vi "AIT 1553 Main Page.vi"(8 "error in (no error)":errorcluster, 11 "Node Ptr":T1 format="%.0x") -> (0 "error out":errorcluster)   [LabVIEW 2015, in "AIT 1553 Custom Device.lvlib"]
uses:
  AIT 1553 Custom Device.lvlib
  <vilib>/NI Veristand/Custom Device API/Custom Device Item Ref.ctl
  Controls and Global/Global.vi
  <vilib>/NI Veristand/Custom Device API/Set Item Property (Boolean).vi
  <vilib>/NI Veristand/Custom Device API/Get Item Property (U16).vi
  <vilib>/NI Veristand/Custom Device API/Get Item Property (Variant).vi
  <vilib>/NI Veristand/Custom Device API/Set Item Property (Variant).vi
  <vilib>/NI Veristand/Custom Device API/Set Item Property (U16).vi
  <vilib>/NI Veristand/Custom Device API/Custom Device API.lvlib
panel:
  in  "Board Index (0 Based)":u16
  in  "Bus 4":bool
  in  "Bus 3":bool
  in  "Bus 2":bool
  in  "Bus 1":bool
  out "Version":string
  in  "Board Serial #":u64
  in  "Header":cluster{"Section Name":string}={"Section Name"="AIT 1553 Device"}
  in  "Description":string
  in  "Name":string
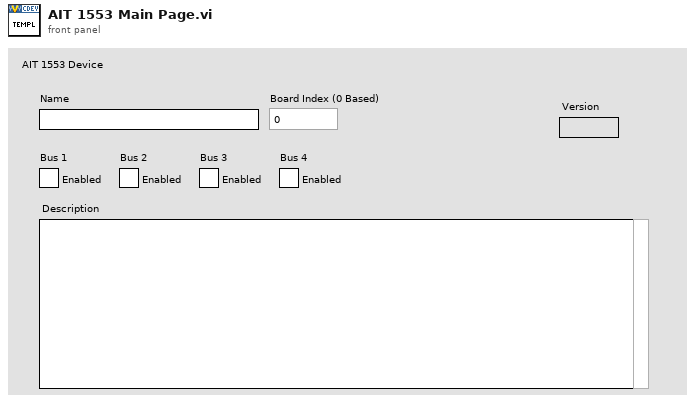
[diagram p1: front panel]
types:
  T1 = typedef "Custom Device API.lvlib/Custom Device Item Ref.ctl" = u64
  T2 = typedef "AIT 1553 Custom Device.lvlib/1553 Bus Enabled.ctl" = cluster{"Bus1Enabled":bool, "Bus2Enabled":bool, "Bus3Enabled":bool, "Bus4Enabled":bool}
  T3 = typedef "Custom Device API.lvlib/Custom Device Item Info.ctl" = cluster{"Name":string, "Is Channel":bool, "GUID":string, "Is Waveform":bool}
  T4 = typedef "Custom Device API.lvlib/Custom Device Commands.ctl" = enum16{"Default", "Item renamed", "Shutdown", "Dynamic button pressed"}
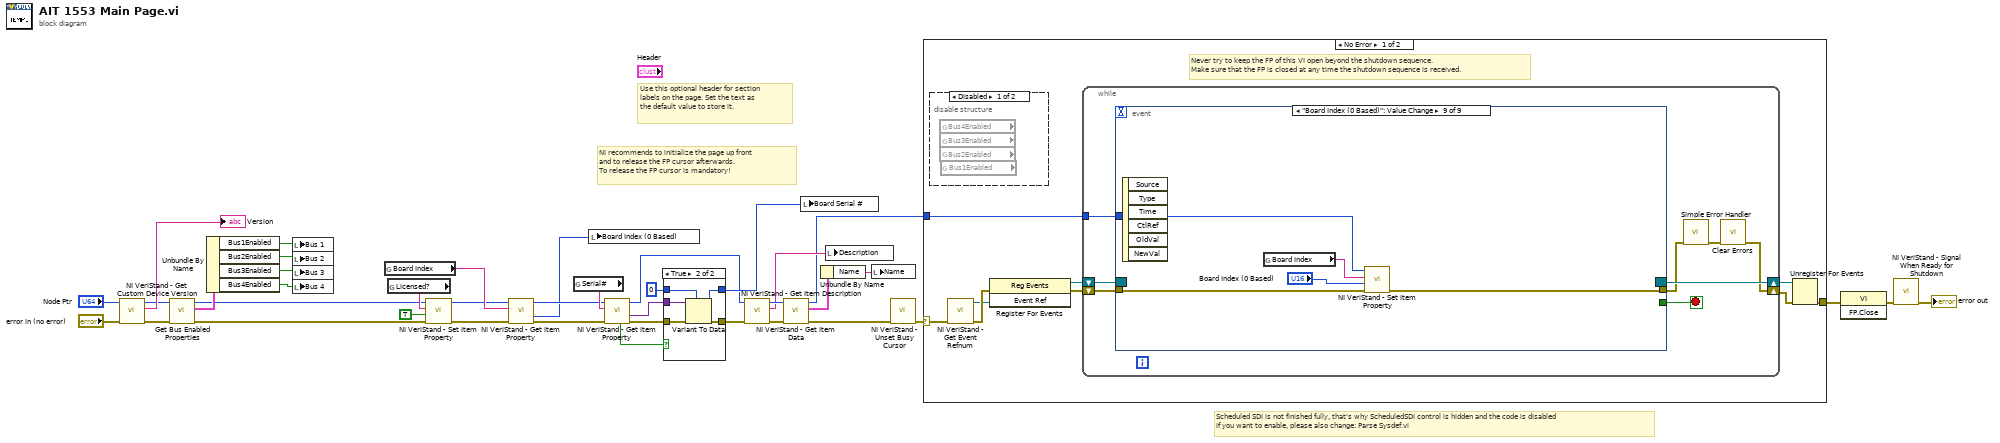
[diagram p0: block diagram]
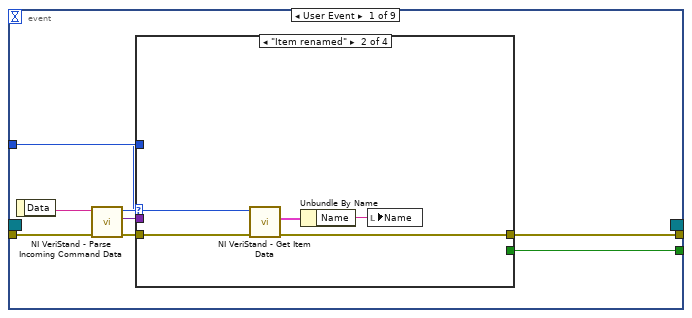
[diagram p4: hidden frame]
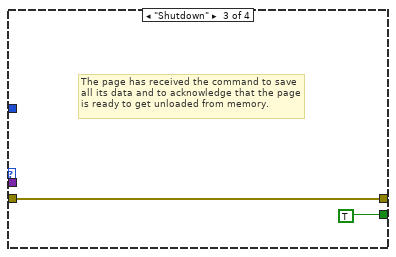
[diagram p6: hidden frame]
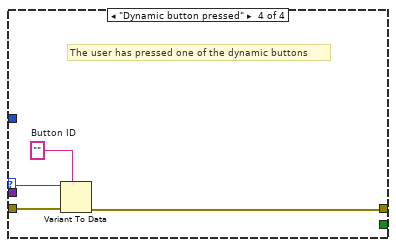
[diagram p7: hidden frame]
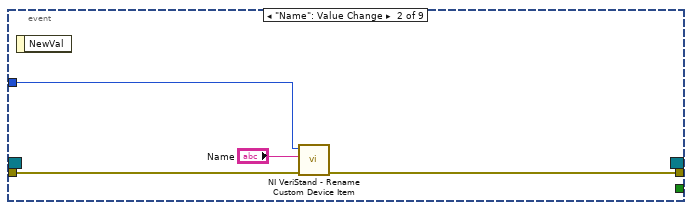
[diagram p8: hidden frame]
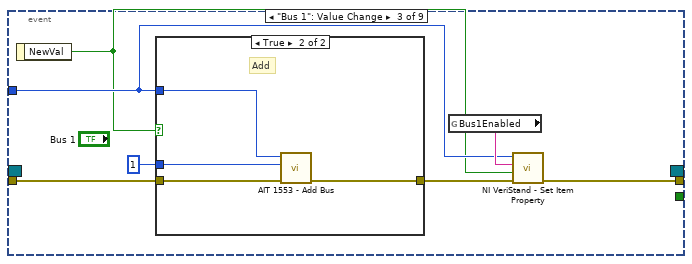
[diagram p9: hidden frame]
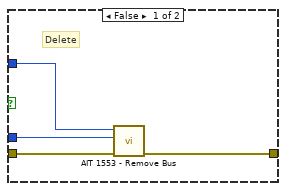
[diagram p10: hidden frame]
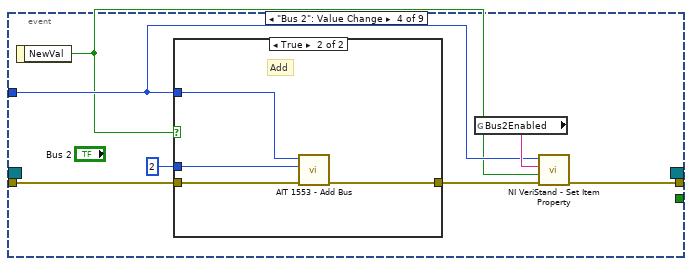
[diagram p11: hidden frame]
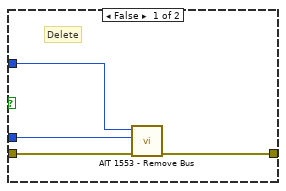
[diagram p12: hidden frame]
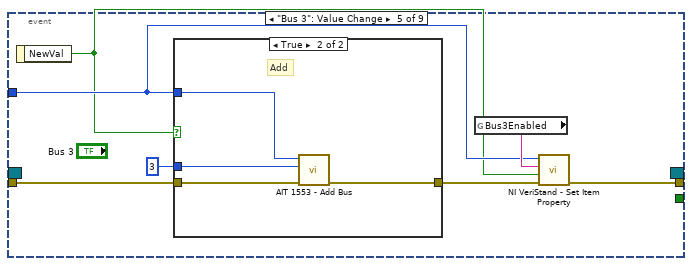
[diagram p13: hidden frame]
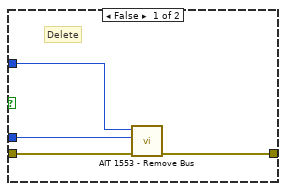
[diagram p14: hidden frame]
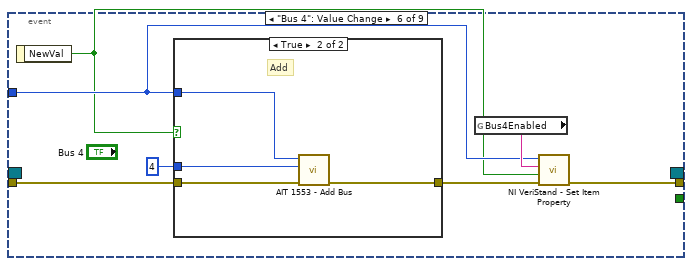
[diagram p15: hidden frame]
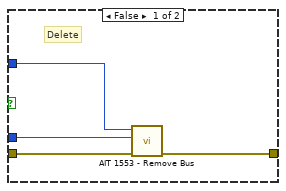
[diagram p16: hidden frame]
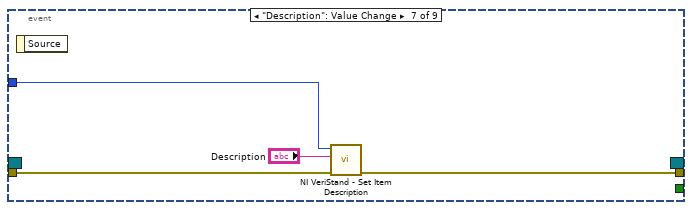
[diagram p17: hidden frame]
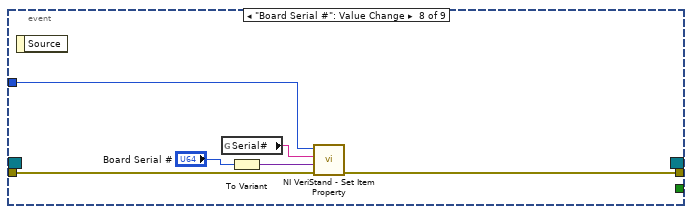
[diagram p18: hidden frame]
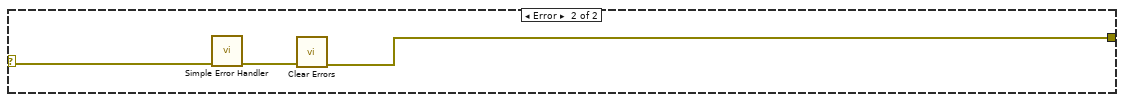
[diagram p19: hidden frame]
diagram:
  # "Scheduled SDI is not finished fully, that's why ScheduledSDI control is hidden and the code is disabled\nIf you want to enable, please also change: Parse Sysdef.vi"
  # "Use this optional header for section labels on the page. Set the text as the default value to store it."
  # "NI recommends to initialize the page up front\nand to release the FP cursor afterwards.\nTo release the FP cursor is mandatory!"
  n1 = call <vilib>:"NI VeriStand - Get Custom Device Version.vi"("error in (no error)"="error in (no error)", "Device Ref in"="Node Ptr") -> ("error out"=w21:errorcluster, "Value"=→"Version":string, "Device Ref out"=w20:T1)  [unwired: 7 in]
  n2 = call "Get Bus Enabled Properties.vi"("error in (no error)"=w21, "Item Ref in"=w20) -> ("error out"=w2:errorcluster, "BusEnabledProperties"=w19:T2, "Item Ref out"=w9:T1)  [unwired: 7 in]
  n3 = Unbundle By Name(w19) -> ("Bus1Enabled"=w18:bool, "Bus2Enabled"=w17:bool, "Bus3Enabled"=w16:bool, "Bus4Enabled"=w15:bool)
  n4 = local write "Bus 1"(w18) -> ()
  n5 = local write "Bus 2"(w17) -> ()
  n6 = local write "Bus 3"(w16) -> ()
  n7 = local write "Bus 4"(w15) -> ()
  n8 = global read "Global.vi" "Board Index"() -> (w7:string)
  n9 = global read "Global.vi" "Licensed?"() -> (w10:string)
  n10 = call-poly <vilib>:"NI VeriStand - Set Item Property.vi"("error in (no error)"=w2, "Value"=TRUE, "Property Name"=w10, "Item Ref in"=w9) -> ("error out"=w8:errorcluster, "Item Ref out"=w6:T1)  [unwired: 5 in, 1 out]
  n11 = call-poly <vilib>:"NI VeriStand - Get Item Property.vi"("error in (no error)"=w8, "Property Name"=w7, "Item Ref in"=w6) -> ("error out"=w4:errorcluster, "Value"=w3:u16, "Item Ref out"=w5:T1)  [unwired: 5 in, 1 out]
  n12 = global read "Global.vi" "Serial#"() -> (w13:string)
  n13 = local write "Board Index (0 Based)"(w3) -> ()
  n14 = call-poly <vilib>:"NI VeriStand - Get Item Property.vi"("error in (no error)"=w4, "Property Name"=w13, "Item Ref in"=w5) -> ("error out"=w28:errorcluster, "Value"=w12:variant, "Item Ref out"=w11:T1, "Found?"=w29:bool)  [unwired: 5 in]
  n15 = case shown="True" w29 {
    tunnel: w28 -> [w40 w46]
    tunnel: [w40 w45] -> w27
    tunnel: u64 0 ("Board Serial #") -> [w41 w44]
    tunnel: [w41 w42] -> w25
    tunnel: w12 -> [_ w43]
    frame False {
    }
    frame True {
      n16 = Variant To Data(error in=w46, type=w44, Variant=w43) -> (data=w42:u64, error out=w45:errorcluster)
    }
  }
  n17 = call <vilib>:"NI VeriStand - Get Item Description.vi"("error in (no error)"=w27, "Item Ref in"=w11) -> ("error out"=w32:errorcluster, "Description"=w33:string, "Item Ref out"=w34:T1)  [unwired: 7 out]
  n18 = call <vilib>:"NI VeriStand - Get Item Data.vi"("error in (no error)"=w32, "Item Ref in"=w34) -> ("error out"=w36:errorcluster, "Item Info"=w31:T3, "Item Ref out"=w14:T1)  [unwired: 7 out]
  n19 = local write "Board Serial #"(w25) -> ()
  n20 = Unbundle By Name(w31) -> ("Name"=w30:string)
  n21 = local write "Description"(w33) -> ()
  n22 = local write "Name"(w30) -> ()
  n23 = call <vilib>:"NI VeriStand - Unset Busy Cursor.vi"("error in (no error)"=w36) -> ("error out"=w35:errorcluster)  [unwired: 10 out]
  n24 = case shown="No Error" w35 {
    selector: w35 -> [w47 w165]
    tunnel: [w52 w163] -> w39
    tunnel: w14 -> [w48 _]
    frame No Error {
      # "Never try to keep the FP of this VI open beyond the shutdown sequence.\nMake sure that the FP is closed at any time the shutdown sequence is received."
      n25 = disable-structure shown="Disabled" {
        frame Disabled {
          n26 = global read "Global.vi" "Bus4Enabled"() -> ()  [unwired: 1 out]
          n27 = global read "Global.vi" "Bus3Enabled"() -> ()  [unwired: 1 out]
          n28 = global read "Global.vi" "Bus2Enabled"() -> ()  [unwired: 1 out]
          n29 = global read "Global.vi" "Bus1Enabled"() -> ()  [unwired: 1 out]
        }
        frame Enabled {
        }
      }
      n30 = call <vilib>:"NI VeriStand - Get Event Refnum.vi"("error in (no error)"=w47) -> ("error out"=w55:errorcluster, "Event Ref"=w51:refnum<user-event>)  [unwired: 9 out]
      n31 = register-events(error in=w55, w51) -> (reference out=w49:refnum<event-registration>, error out=w50:errorcluster)  [unwired: 1 in]
      n32 = while {
        tunnel: w48 -> [w59]
        shift-right: [w56] -> w53
        shift-left: w50 -> [w62]
        shift-right: [w63] -> w54
        shift-left: w49 -> [w61]
        stop <- w60 stop-if-true
        n33 = event shown="[8] \"Board Index (0 Based)\": Value Change" {
          selector: w61 -> [_ _ _ _ _ _ _ _ _]
          dyn-events: [_ _ _ _ _ _ _ _ _] -> w63
          timeout: _ -> [_ _ _ _ _ _ _ _ _]
          tunnel: w62 -> [w71 w87 w94 w109 w124 w139 w150 w157 w162]
          tunnel: [w67 _ _ _ _ _ _ _ _] -> w60
          tunnel: [w66 w86 w92 w104 w119 w134 w149 w156 w161] -> w58
          tunnel: w59 -> [w65 w85 w90 w106 w121 w136 w151 w153 w159]
          event User Event {
            n34 = event-data() -> ("Data"=w70:string)  [unwired: 1 out]
            n35 = call <vilib>:"NI VeriStand - Parse Incoming Command Data.vi"("error in (no error)"=w71, "Incoming data"=w70) -> ("error out"=w69:errorcluster, "Outgoing data"=w64:variant, "Action"=w68:T4)  [unwired: 7 out]
            n36 = case shown="\"Item renamed\"" w68 {
              tunnel: w69 -> [w72 w77 w78 w83]
              tunnel: [_ _ TRUE _] -> w67
              tunnel: [w72 w74 w78 w80] -> w66
              tunnel: w65 -> [_ w76 _ _]
              tunnel: w64 -> [_ _ _ w82]
              frame "Default", Default {
              }
              frame "Item renamed" {
                n37 = call <vilib>:"NI VeriStand - Get Item Data.vi"("error in (no error)"=w77, "Item Ref in"=w76) -> ("error out"=w74:errorcluster, "Item Info"=w75:T3)  [unwired: 8 out]
                n38 = Unbundle By Name(w75) -> ("Name"=w73:string)
                n39 = local write "Name"(w73) -> ()
              }
              frame "Shutdown" {
                # "The page has received the command to save all its data and to acknowledge that the page is ready to get unloaded from memory."
              }
              frame "Dynamic button pressed" {
                w81 = ""  # Button ID
                # "The user has pressed one of the dynamic buttons"
                n40 = Variant To Data(error in=w83, type=w81, Variant=w82) -> (error out=w80:errorcluster)  [unwired: 1 out]
              }
            }
          }
          event "Name": Value Change {
            n41 = event-data() -> ()  [unwired: 2 out]
            n42 = call <vilib>:"NI VeriStand - Rename Custom Device Item.vi"("error in (no error)"=w87, "New Name"="Name", "Item Ref in"=w85) -> ("error out"=w86:errorcluster)  [unwired: 1 in, 7 out]
          }
          event "Bus 1": Value Change {
            n43 = event-data() -> ("NewVal"=w89:bool)  [unwired: 1 out]
            n44 = case shown="True" w89 {
              tunnel: w94 -> [w98 w102]
              tunnel: [w95 w101] -> w93
              tunnel: w90 -> [w97 w100]
              tunnel: u16 1 ("Bus") -> [w96 w99]
              frame False {
                # "Delete"
                n45 = call "AIT 1553 - Remove Bus.vi"("error in (no error)"=w98, "Bus"=w96, "Node Ptr"=w97) -> ("error out"=w95:errorcluster)  [unwired: 8 in]
              }
              frame True {
                # "Add"
                n46 = call "AIT 1553 - Add Bus.vi"("error in (no error)"=w102, "Bus"=w99, "Node Ptr"=w100) -> ("error out"=w101:errorcluster)  [unwired: 7 in, 1 out]
              }
            }
            n47 = global read "Global.vi" "Bus1Enabled"() -> (w91:string)
            n48 = call-poly <vilib>:"NI VeriStand - Set Item Property.vi"("error in (no error)"=w93, "Value"=w89, "Property Name"=w91, "Item Ref in"=w90) -> ("error out"=w92:errorcluster)  [unwired: 5 in, 2 out]
          }
          event "Bus 2": Value Change {
            n49 = event-data() -> ("NewVal"=w105:bool)  [unwired: 1 out]
            n50 = case shown="True" w105 {
              tunnel: w109 -> [w113 w117]
              tunnel: [w112 w116] -> w107
              tunnel: w106 -> [w111 w115]
              tunnel: u16 2 ("Bus") -> [w110 w114]
              frame False {
                # "Delete"
                n51 = call "AIT 1553 - Remove Bus.vi"("error in (no error)"=w113, "Bus"=w110, "Node Ptr"=w111) -> ("error out"=w112:errorcluster)  [unwired: 8 in]
              }
              frame True {
                # "Add"
                n52 = call "AIT 1553 - Add Bus.vi"("error in (no error)"=w117, "Bus"=w114, "Node Ptr"=w115) -> ("error out"=w116:errorcluster)  [unwired: 7 in, 1 out]
              }
            }
            n53 = global read "Global.vi" "Bus2Enabled"() -> (w108:string)
            n54 = call-poly <vilib>:"NI VeriStand - Set Item Property.vi"("error in (no error)"=w107, "Value"=w105, "Property Name"=w108, "Item Ref in"=w106) -> ("error out"=w104:errorcluster)  [unwired: 5 in, 2 out]
          }
          event "Bus 3": Value Change {
            n55 = event-data() -> ("NewVal"=w120:bool)  [unwired: 1 out]
            n56 = case shown="True" w120 {
              tunnel: w124 -> [w128 w132]
              tunnel: [w127 w131] -> w122
              tunnel: w121 -> [w126 w130]
              tunnel: u16 3 ("Bus") -> [w125 w129]
              frame False {
                # "Delete"
                n57 = call "AIT 1553 - Remove Bus.vi"("error in (no error)"=w128, "Bus"=w125, "Node Ptr"=w126) -> ("error out"=w127:errorcluster)  [unwired: 8 in]
              }
              frame True {
                # "Add"
                n58 = call "AIT 1553 - Add Bus.vi"("error in (no error)"=w132, "Bus"=w129, "Node Ptr"=w130) -> ("error out"=w131:errorcluster)  [unwired: 7 in, 1 out]
              }
            }
            n59 = global read "Global.vi" "Bus3Enabled"() -> (w123:string)
            n60 = call-poly <vilib>:"NI VeriStand - Set Item Property.vi"("error in (no error)"=w122, "Value"=w120, "Property Name"=w123, "Item Ref in"=w121) -> ("error out"=w119:errorcluster)  [unwired: 5 in, 2 out]
          }
          event "Bus 4": Value Change {
            n61 = event-data() -> ("NewVal"=w135:bool)  [unwired: 1 out]
            n62 = case shown="True" w135 {
              tunnel: w139 -> [w143 w147]
              tunnel: [w142 w146] -> w137
              tunnel: w136 -> [w141 w145]
              tunnel: u16 4 ("Bus") -> [w140 w144]
              frame False {
                # "Delete"
                n63 = call "AIT 1553 - Remove Bus.vi"("error in (no error)"=w143, "Bus"=w140, "Node Ptr"=w141) -> ("error out"=w142:errorcluster)  [unwired: 8 in]
              }
              frame True {
                # "Add"
                n64 = call "AIT 1553 - Add Bus.vi"("error in (no error)"=w147, "Bus"=w144, "Node Ptr"=w145) -> ("error out"=w146:errorcluster)  [unwired: 7 in, 1 out]
              }
            }
            n65 = global read "Global.vi" "Bus4Enabled"() -> (w138:string)
            n66 = call-poly <vilib>:"NI VeriStand - Set Item Property.vi"("error in (no error)"=w137, "Value"=w135, "Property Name"=w138, "Item Ref in"=w136) -> ("error out"=w134:errorcluster)  [unwired: 5 in, 2 out]
          }
          event "Description": Value Change {
            n67 = event-data() -> ()  [unwired: 2 out]
            n68 = call <vilib>:"NI VeriStand - Set Item Description.vi"("error in (no error)"=w150, "Description"="Description", "Item Ref in"=w151) -> ("error out"=w149:errorcluster)  [unwired: 8 out]
          }
          event "Board Serial #": Value Change {
            n69 = event-data() -> ()  [unwired: 2 out]
            n70 = global read "Global.vi" "Serial#"() -> (w154:string)
            n71 = To Variant(anything="Board Serial #") -> (Variant=w155:variant)
            n72 = call-poly <vilib>:"NI VeriStand - Set Item Property.vi"("error in (no error)"=w157, "Value"=w155, "Property Name"=w154, "Item Ref in"=w153) -> ("error out"=w156:errorcluster)  [unwired: 5 in, 2 out]
          }
          event "Board Index (0 Based)": Value Change {
            n73 = event-data() -> ()  [unwired: 7 out]
            n74 = global read "Global.vi" "Board Index"() -> (w160:string)
            n75 = call-poly <vilib>:"NI VeriStand - Set Item Property.vi"("error in (no error)"=w162, "Value"="Board Index (0 Based)", "Property Name"=w160, "Item Ref in"=w159) -> ("error out"=w161:errorcluster)  [unwired: 5 in, 2 out]
          }
        }
        n76 = call <vilib>:"Simple Error Handler.vi"("error in (no error)"=w58) -> ("error out"=w57:errorcluster)  [unwired: 1 in, 7 out]
        n77 = call <vilib>:"Clear Errors.vi"("error in (no error)"=w57) -> ("error out"=w56:errorcluster)  [unwired: 1 in, 5 out]
      }
      n78 = Unregister For Events(event registration refnum=w54, error in=w53) -> (error out=w52:errorcluster)
    }
    frame Error {
      n79 = call <vilib>:"Simple Error Handler.vi"("error in (no error)"=w165) -> ("error out"=w164:errorcluster)  [unwired: 1 in, 7 out]
      n80 = call <vilib>:"Clear Errors.vi"("error in (no error)"=w164) -> ("error out"=w163:errorcluster)  [unwired: 1 in, 5 out]
    }
  }
  n81 = invoke class="VI" method="FP.Close"(error in=w39) -> (error out=w38:errorcluster)  [unwired: 2 in, 2 out]
  n82 = call <vilib>:"NI VeriStand - Signal When Ready for Shutdown.vi"("error in (no error)"=w38) -> ("error out"=→"error out":errorcluster)  [unwired: 10 out]
